vi "program seq..vi"(6 "IOList":T3, 7 "Cluster data":T5, 11 "Filepath":path=path "E:/My Project/2018-2019/Under development/Minda Ind. Switch -ID 144-145/Project/data/trail pro -12.txt") -> (0 "Error Out":errorcluster)   [LabVIEW 2015]
uses:
  Control PB/Active.ctl
  Control PB/deactive.ctl
  Control PB/output control.ctl
  Control PB/input control.ctl
  Control PB/timer.ctl
  Control PB/Remove list.ctl
  Control Button/Exit.ctl
  Control PB/Add_s.ctl
  Control PB/Delete_.ctl
  Control Button/Save.ctl
  Control PB/motor.ctl
  Control PB/Camera.ctl
  Control PB/Barcode.ctl
  Galobal variable_TI.vi
panel:
  in  "CAN":bool
  in  "Feature Step edit":bool
  out "Step List 4":string[](array[string])
  out "Step List 3":string[](array[string])
  in  "Barcode":T1
  in  "Camera":T2
  out "x <= y?":bool
  out "Cancel":bool
  out "Step List 2":string[](array[string])
  out "Pokayoka Result":cluster{"Sensor Name":string, "Boolean":bool}[](array[cluster])
  in  "Feed Back Channel":i32[](listbox)=[0]
  out "Input":bool[](array[boolean])
  out "Feature List (Out) 2":T4(array[cluster])
  out "error out 2":errorcluster
  in  "Control":bool
  out "Station No":string
  out "Model Name":string
  out "Model":string
  in  "Motor":T6
  in  "Feature List":i32(listbox) caption="Steps List"
  in  "Deletefeature list":T7
  in  "Add feature list":T8
  in  "Deactive":T9
  in  "Active":T10
  in  "Program step":i32(listbox)
  in  "Remove Step":T11
  in  "Wait Time":u32=100 caption="Timer(ms)" max=600000 step=1
  in  "Timer":T12
  in  "Save":T13
  in  "stop":T14
  in  "op Add":T15
  in  "Input Add":T16
  out "Step List":string[](array[string])
  out "output cluster":T17
  in  "Analog":bool
  in  "Analog Input":i32[](listbox)=[0]
  in  "Control Channel":i32[](listbox)=[7]
  in  "Steps":T18(array[cluster])
  in  "Program mode":string="Data"
  out "error out":errorcluster
  out "Feature List (Out)":T19(array[cluster])
  # "Program Sequence Window"
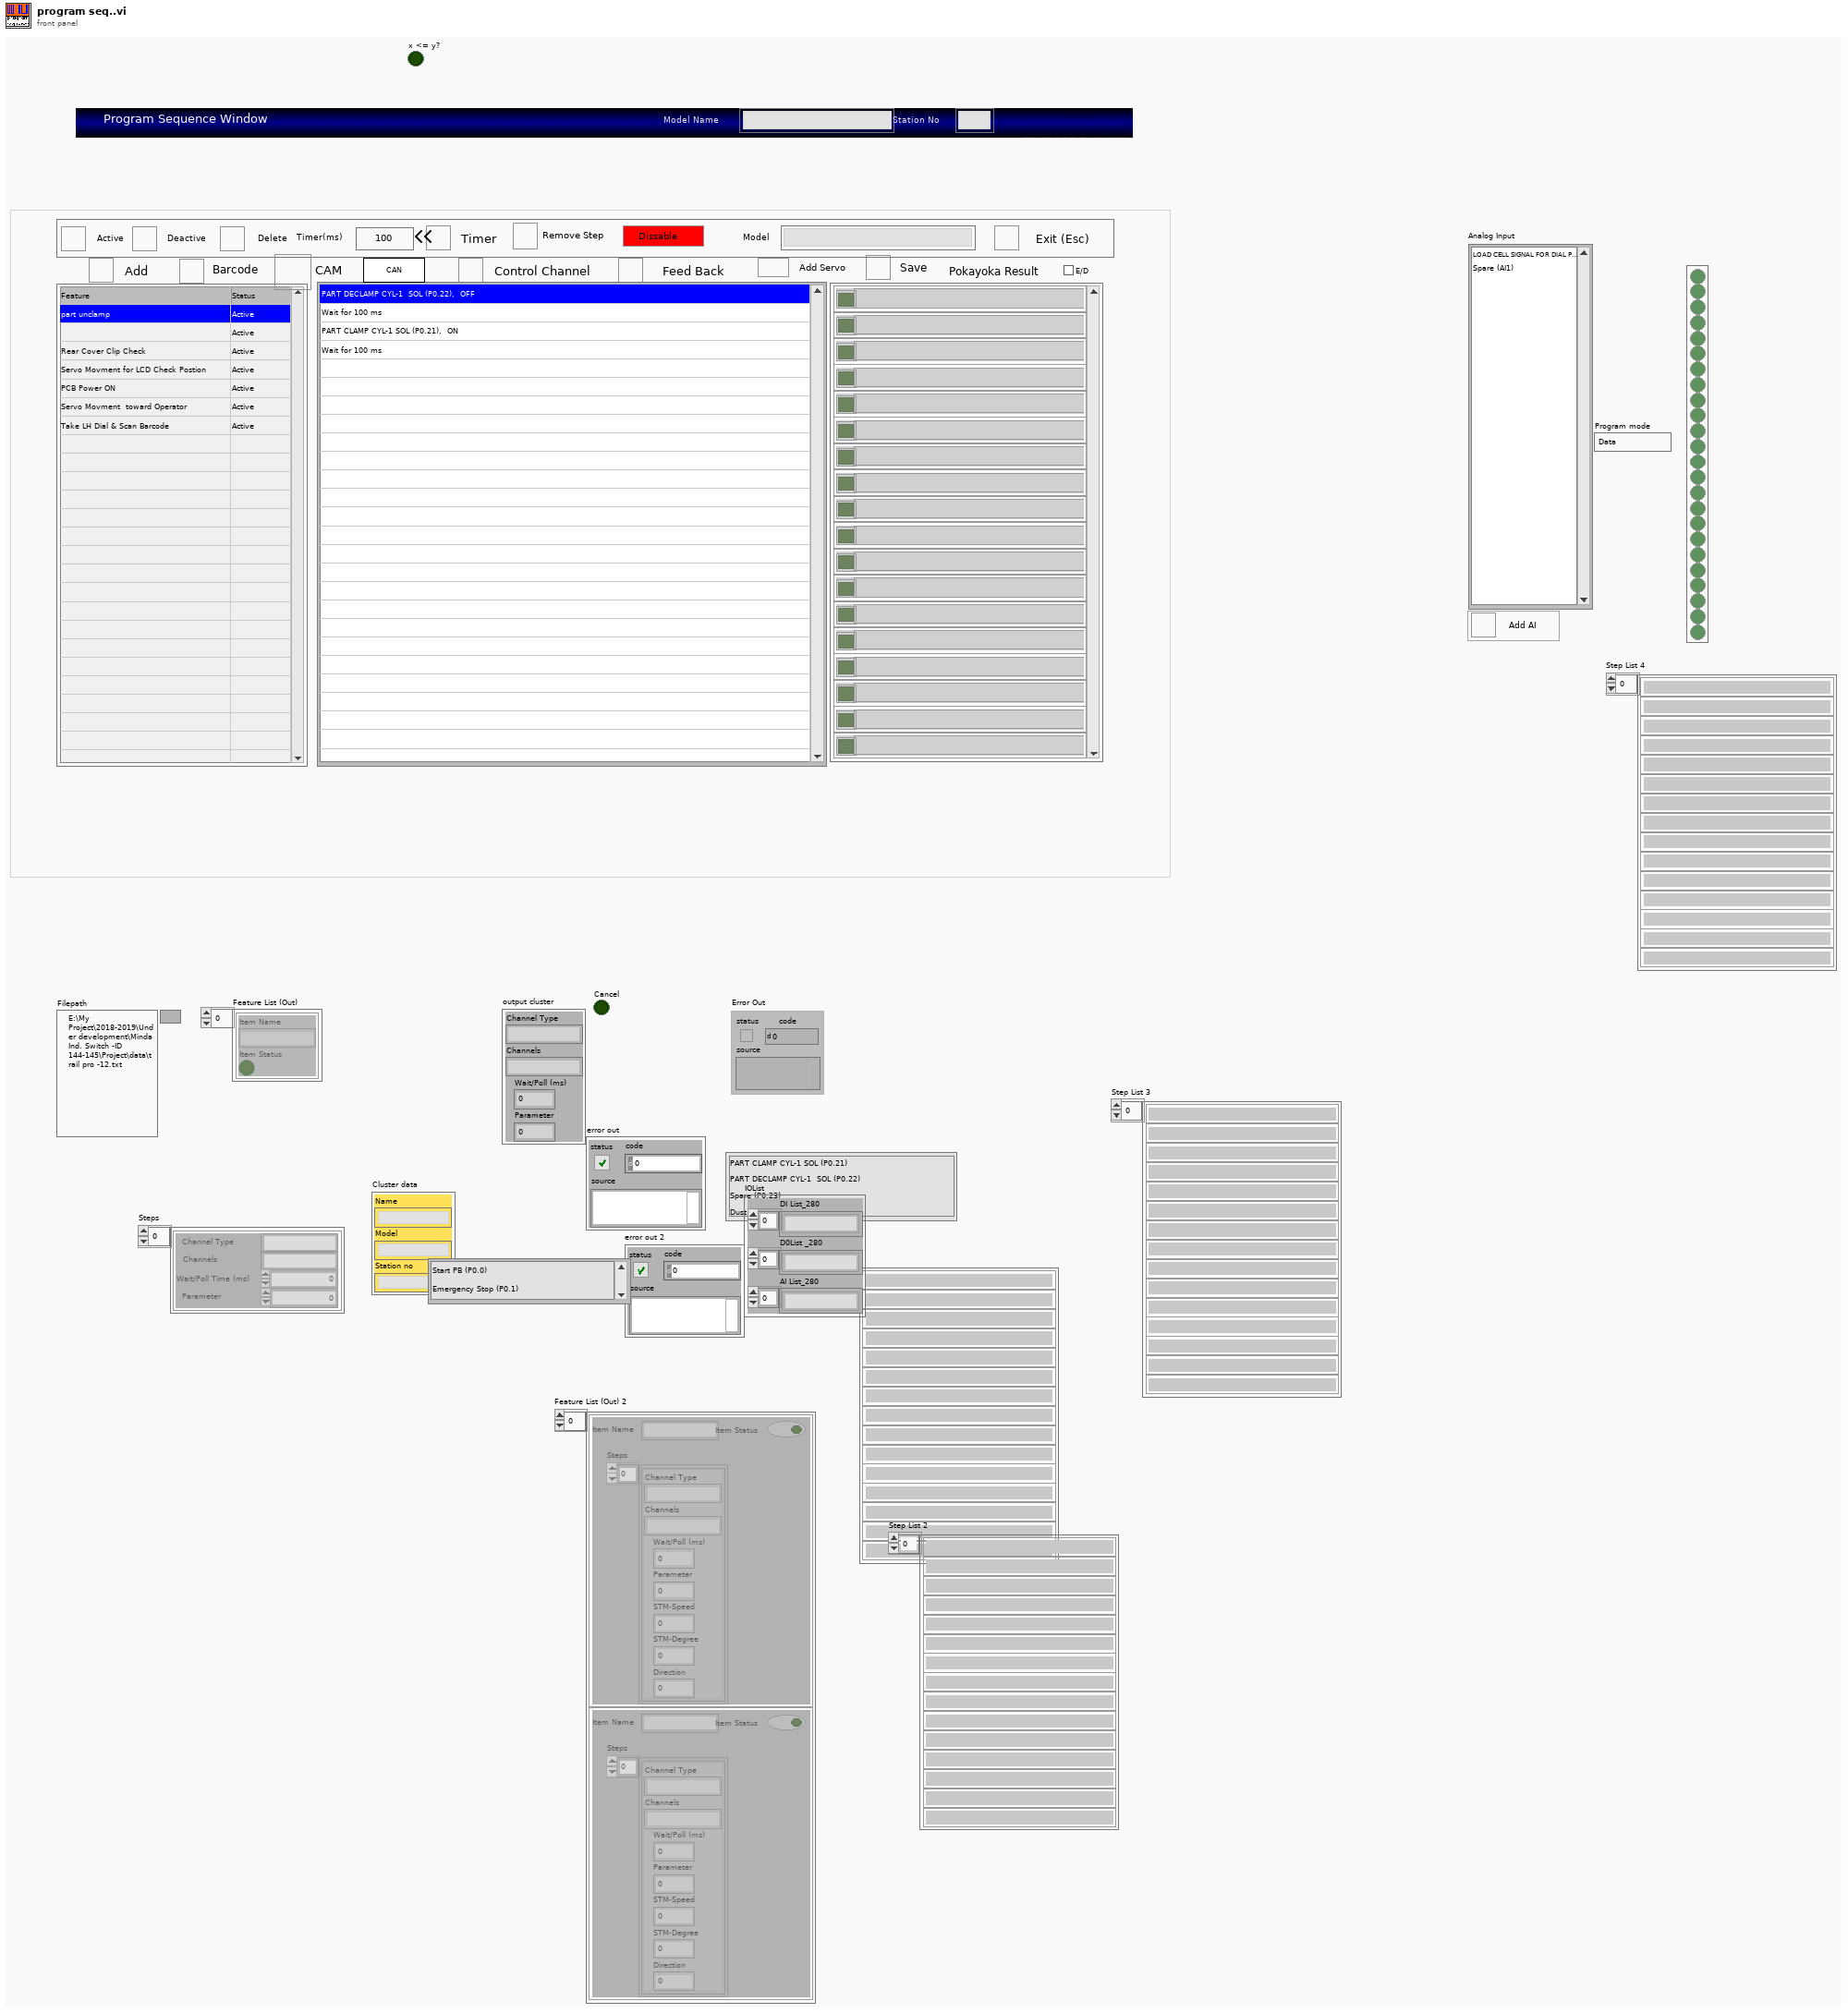
[diagram p1: front panel]
types:
  T1 = typedef "Barcode.ctl" = bool
  T2 = typedef "Camera.ctl" = bool
  T3 = cluster{"DI List_280":string[], "D0List _280":string[], "AI List_280":string[]}
  T4 = cluster{"Item Name":string, "Item Status":bool, "Steps":cluster{"Channel Type":string, "Channels":string, "Wait/Poll (ms)":u32, "Parameter":u8, "STM-Speed":i32, "STM-Degree":u32, "Direction":u8}[]}[]
  T5 = cluster{"Name":string, "Model":string, "Station no":string}
  T6 = typedef "motor.ctl" = bool
  T7 = typedef "Delete_.ctl" = bool
  T8 = typedef "Add_s.ctl" = bool
  T9 = typedef "deactive.ctl" = bool
  T10 = typedef "Active.ctl" = bool
  T11 = typedef "Remove list.ctl" = bool
  T12 = typedef "timer.ctl" = bool
  T13 = typedef "Save.ctl" = bool
  T14 = typedef "Exit.ctl" = bool
  T15 = typedef "output control.ctl" = bool
  T16 = typedef "input control.ctl" = bool
  T17 = cluster{"Channel Type":string, "Channels":string, "Wait/Poll (ms)":u32, "Parameter":u8}
  T18 = cluster{"Channel Type":string, "Channels":string, "Wait/Poll Time (ms)":u32, "Parameter":u8}[]
  T19 = cluster{"Item Name":string, "Item Status":bool}[]
  T20 = cluster{"Channel Type":string, "Channels":string, "Wait/Poll (ms)":u32, "Parameter":u8, "STM-Speed":i32, "STM-Degree":i32, "Direction":u8}
  T21 = cluster{"Item Name":string, "Item Status":bool, "Steps":cluster{"Channel Type":string, "Channels":string, "Wait/Poll (ms)":u32, "Parameter":u8, "STM-Speed":i32, "STM-Degree":u32, "Direction":u8}[]}
  T22 = cluster{"Channel Type":string, "Channels":string, "Wait/Poll (ms)":u32, "Parameter":u8, "STM-Speed":i32, "STM-Degree":u32, "Direction":u8}[]
  T23 = cluster{"Item Name":string, "Active":T10, "Steps":cluster{"Channel Type":string, "Channels":string, "Wait/Poll (ms)":u32, "Parameter":u8, "STM-Speed":i32, "STM-Degree":u32, "Direction":u8}[]}
  T24 = cluster{"Channel Type":string, "Channels":string, "Wait/Poll (ms)":u32, "Parameter":u8, "STM-Speed":i32, "STM-Degree":i32, "Direction":u8}[]
  T25 = cluster{"Feature name ":string, bool, cluster{"Channel Type":string, "Channels":string, "Wait/Poll (ms)":u32, "Parameter":u8, "STM-Speed":i32, "STM-Degree":i32, "Direction":u8}[]}
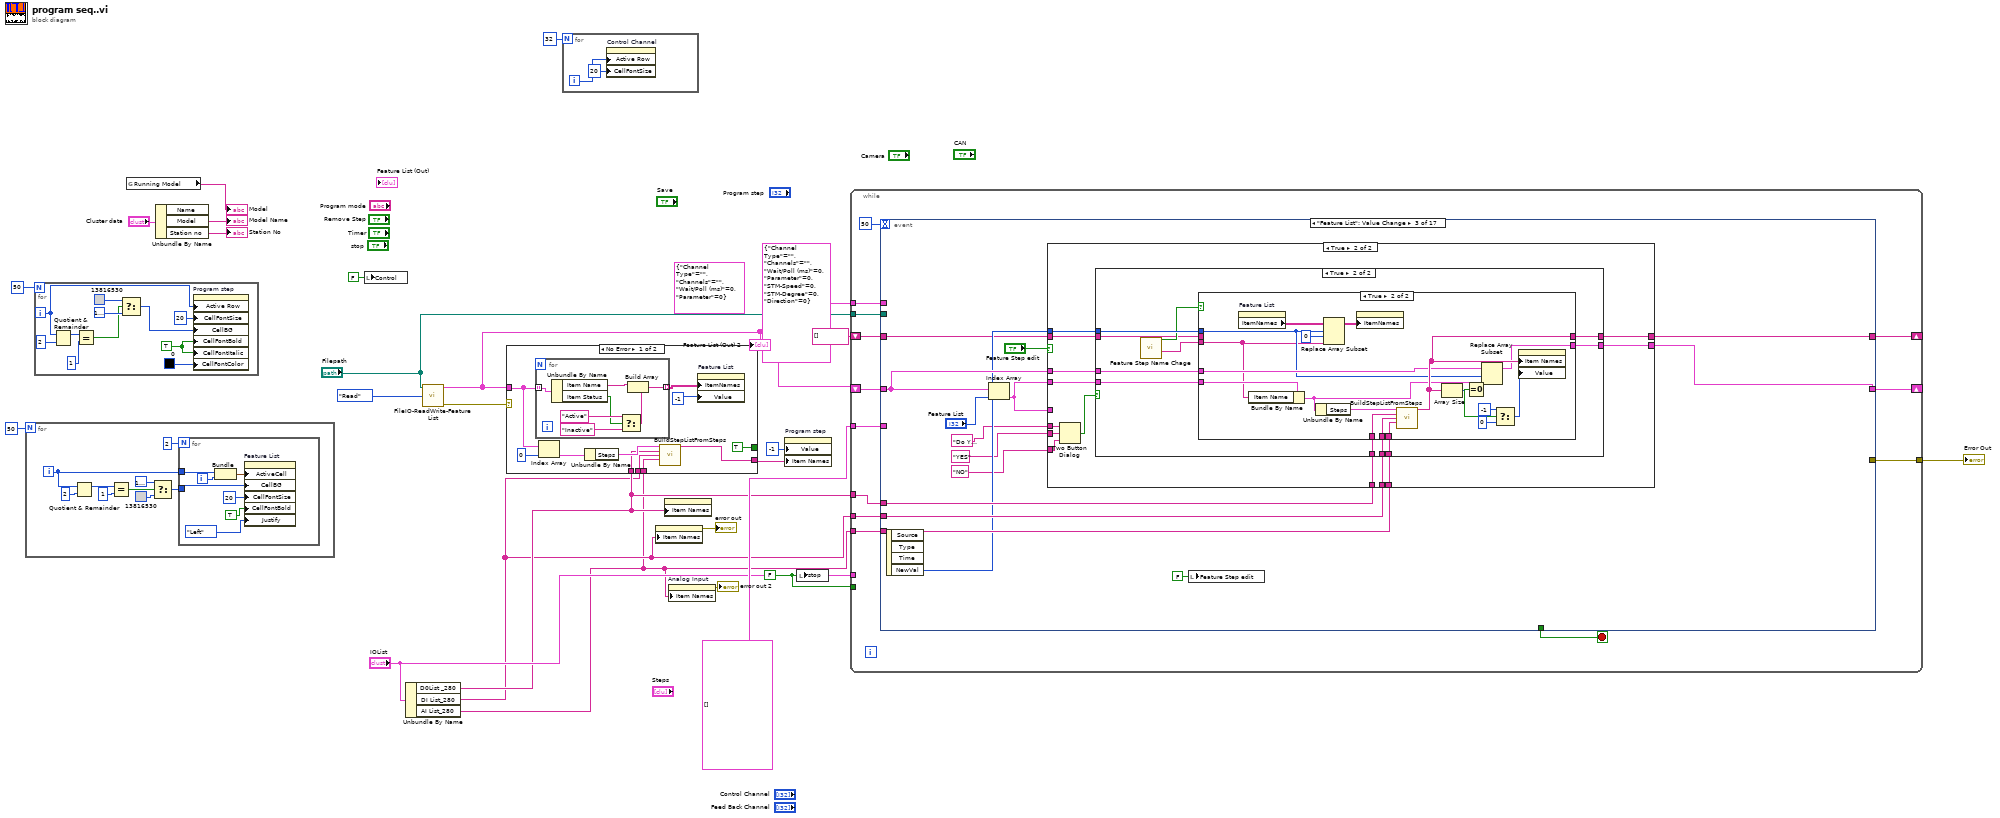
[diagram p0: block diagram]
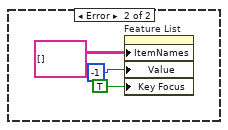
[diagram p2: hidden frame]
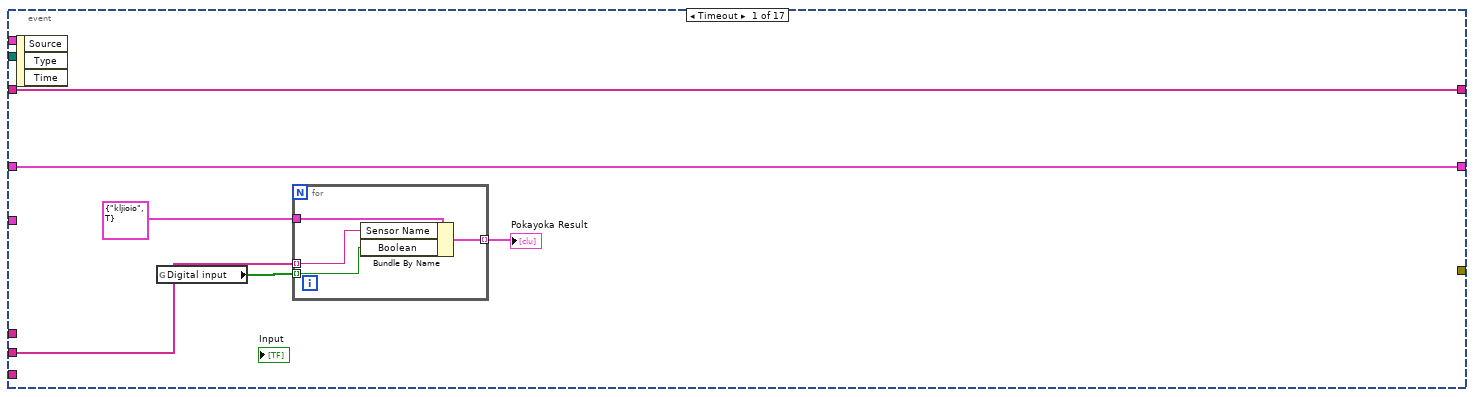
[diagram p3: hidden frame]
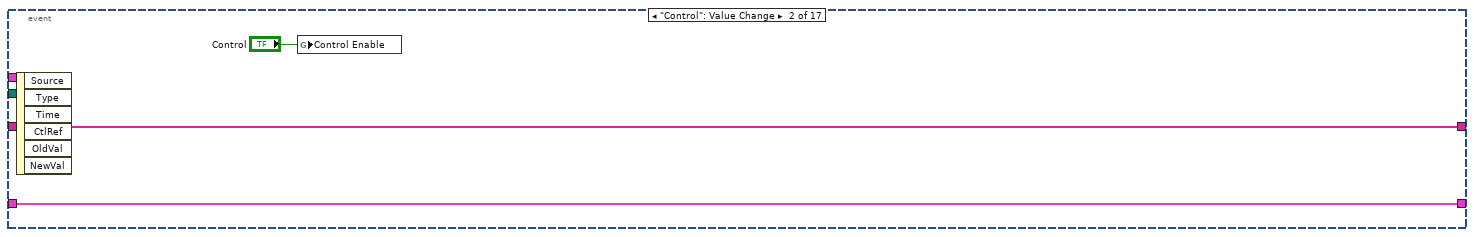
[diagram p4: hidden frame]
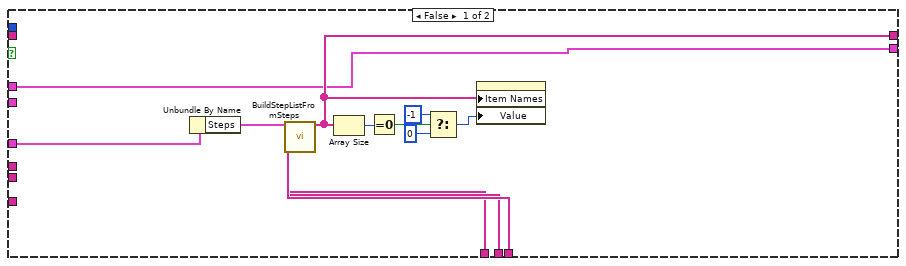
[diagram p5: hidden frame]
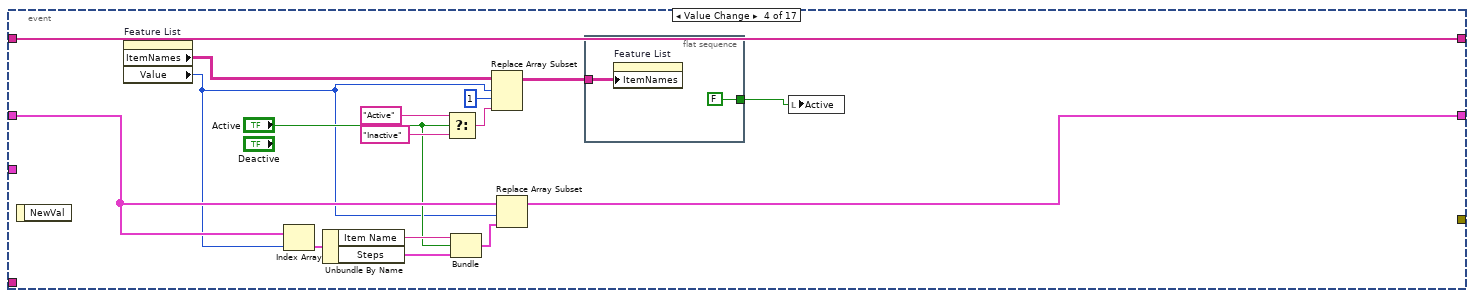
[diagram p8: hidden frame]
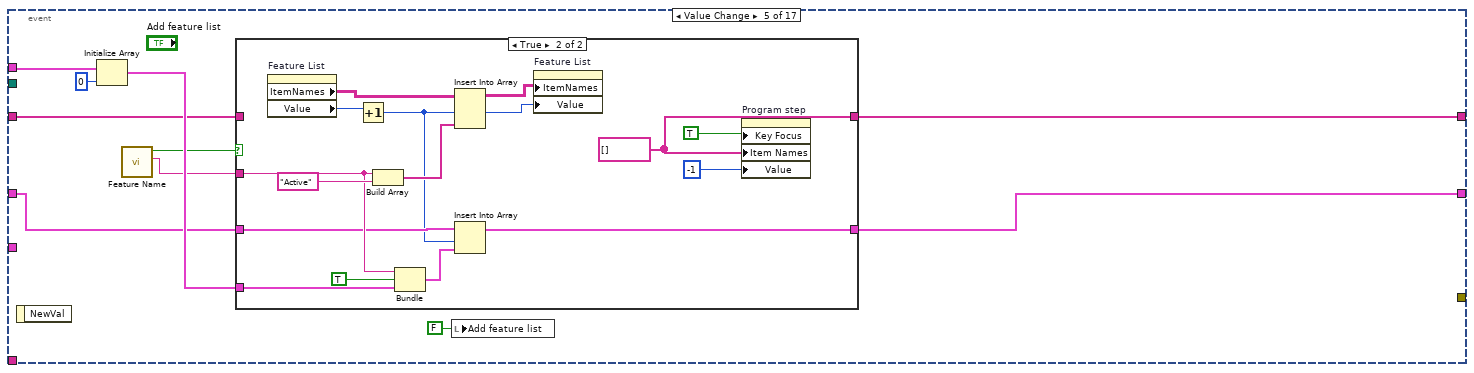
[diagram p9: hidden frame]
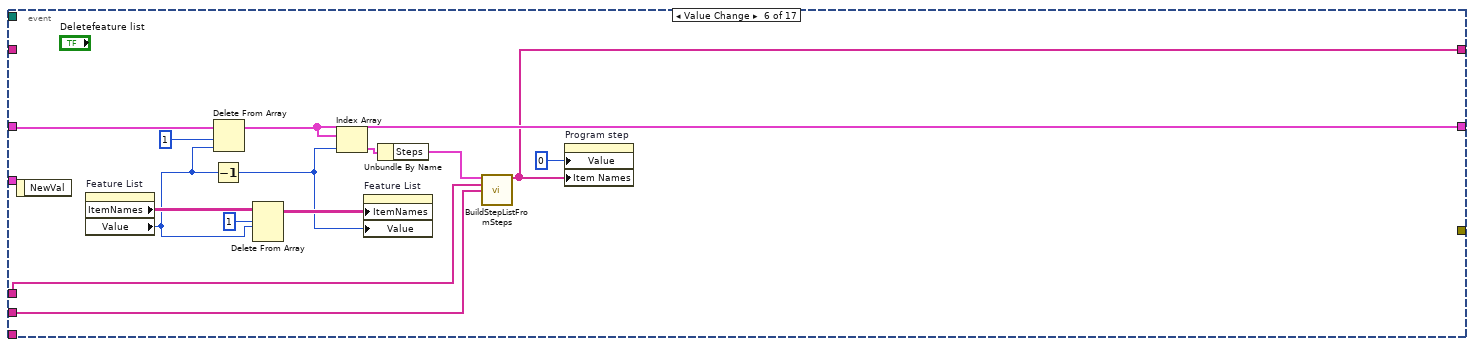
[diagram p11: hidden frame]
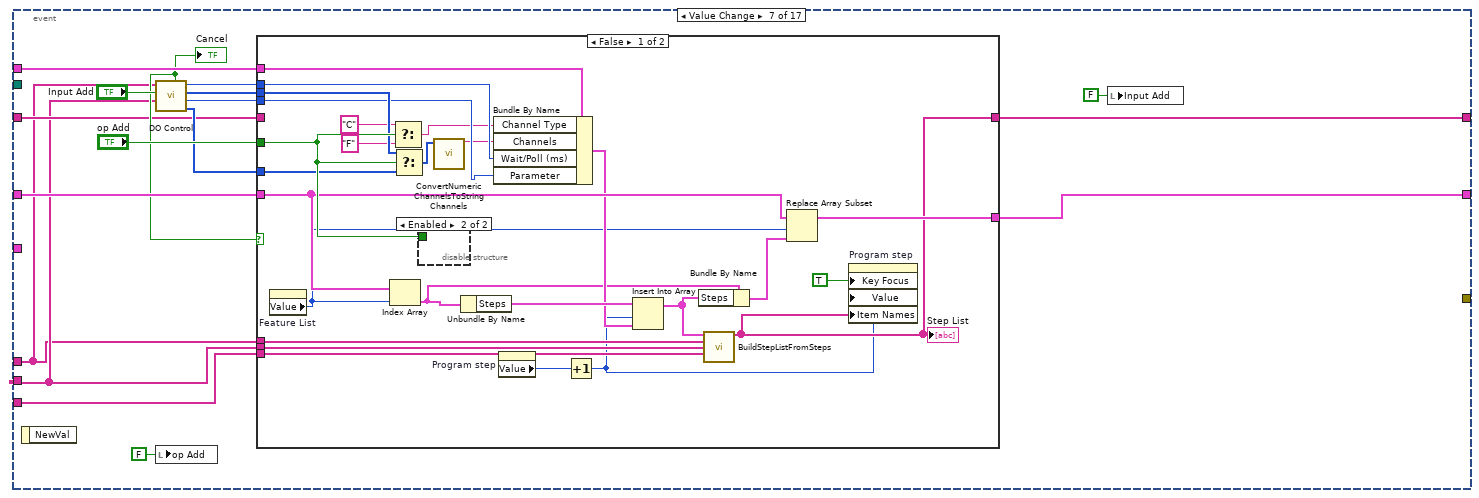
[diagram p12: hidden frame]
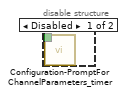
[diagram p13: hidden frame]
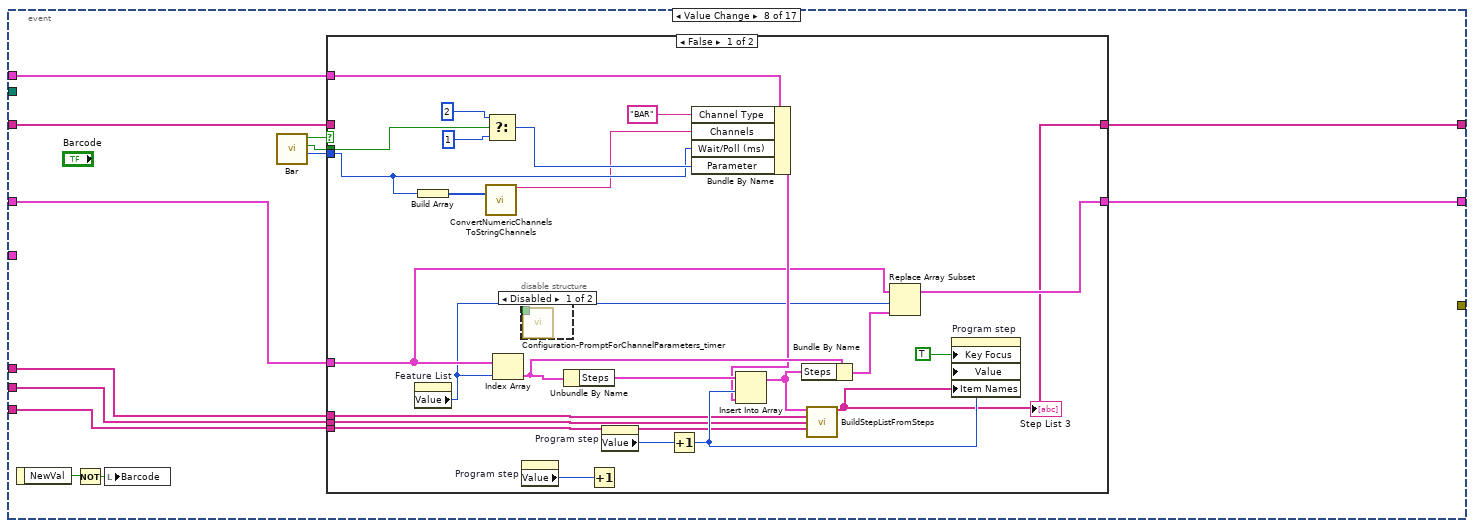
[diagram p15: hidden frame]
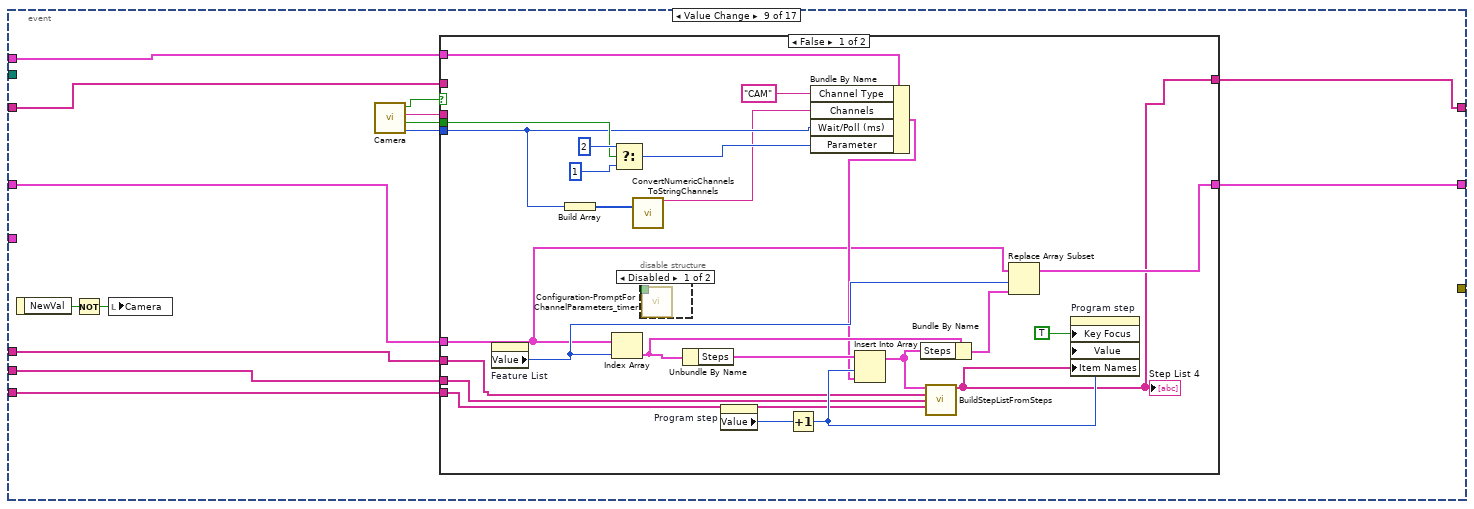
[diagram p18: hidden frame]
diagram:
  w9 = FALSE ("stop")
  (unwired) T17 {"Channel Type"="", "Channels"="", "Wait/Poll (ms)"=0, "Parameter"=0} ("Step")
  n1 = for {
    N: 50 -> [_]
    i -> [w33]
    n2 = Quotient & Remainder(x=w33, y=2) -> (x-y*floor(x/y)=w31:i32)  [unwired: 1 out]
    n3 = Equal?(x=w31, y=1) -> (x = y?=w29:bool)
    n4 = Select(t=u32 16777225 ("Color Box"), s=w29, f=u32 13816530 ("Color Box")) -> (s? t:f=w26:u32)
    n5 = for {
      N: 2 -> [_]
      tunnel: w33 -> [w41]
      tunnel: w26 -> [w38]
      i -> [w40]
      n6 = Bundle(w41, w40) -> (w39:cluster{i32, i32})  [unwired: 1 in]
      n7 = property on="Feature List" class="MCListbox (strict)"("ActiveCell"=w39, "CellBG"=w38, "CellFontSize"=u32 20 ("Active Cell:Cell Font:Size"), "CellFontBold"=TRUE ("Active Cell:Cell Font:Bold"), "Justify"=enum16{"Left", "Center", "Right"}."Left" ("Active Cell:Cell Justification")) -> ()  [unwired: 2 in, 2 out]
    }
  }
  n8 = for {
    N: 50 -> [_]
    i -> [w46]
    w43 = TRUE
    n9 = Quotient & Remainder(x=w46, y=2) -> (x-y*floor(x/y)=w49:i32)  [unwired: 1 out]
    n10 = Equal?(x=w49, y=1) -> (x = y?=w47:bool)
    n11 = Select(t=u32 13816530 ("Color Box"), s=w47, f=u32 16777226 ("Color Box")) -> (s? t:f=w44:u32)
    n12 = property on="Program step" class="LstBox (strict)"("Active Row"=w46, "CellFontSize"=u32 20 ("Active Row:Cell Font:Size"), "CellBG"=w44, "CellFontBold"=w43, "CellFontItalic"=w43, "CellFontColor"=u32 0 ("Color Box")) -> ()  [unwired: 2 in, 2 out]
  }
  n13 = global read "Galobal variable_TI.vi" "Running Model"() -> (→"Model":string)
  n14 = Unbundle By Name("Cluster data") -> ("Model"=→"Model Name":string, "Station no"=→"Station No":string)  [unwired: 1 out]
  n15 = local write "Control"(FALSE ("Control")) -> ()
  n16 = Unbundle By Name("IOList") -> ("D0List _280"=w5:string[], "DI List_280"=w4:string[], "AI List_280"=w3:string[])
  n17 = call "FileIO-ReadWrite-FeatureList.vi"("Filepath"="Filepath", "Read/Write"=enum16{"Read", "Write"}."Read") -> ("Feature List (Out)"=w16:T4, "Error Out"=w20:errorcluster)  [unwired: 12 in]
  "Feature List (Out) 2" <- w16
  n18 = case shown="No Error" w20 {
    tunnel: w16 -> [w63 _]
    tunnel: w5 -> [w59 _]
    tunnel: w4 -> [w58 _]
    tunnel: w3 -> [w57 _]
    tunnel: [w56 _] -> w19
    tunnel: [TRUE ("Key Focus") _] -> _
    frame No Error {
      n19 = for {
        tunnel: w63 -> [w70] mode=indexing
        tunnel: [w64] -> w54 mode=indexing
        n20 = Unbundle By Name(w70) -> ("Item Name"=w66:string, "Item Status"=w67:bool)
        n21 = Select(t="Active", s=w67, f="Inactive") -> (s? t:f=w65:string)
        n22 = Build Array(w66, w65) -> (w64:string[])
      }
      n23 = Index Array(array=w63, index=0) -> (element=w61:T21)
      n24 = Unbundle By Name(w61) -> ("Steps"=w60:T22)
      n25 = call "BuildStepListFromSteps.vi"("Steps"=w60, "Control Channels"=w59, "Feedback Channels"=w58, "AI"=w57) -> ("Step List"=w56:string[])  [unwired: 11 in]
      n26 = property on="Feature List" class="MCListbox (strict)"("ItemNames"=w54, "Value"=-1 ("Feautre list")) -> ()  [unwired: 2 in, 2 out]
    }
    frame Error {
      n27 = property on="Feature List" class="MCListbox (strict)"("ItemNames"=string[][] [] ("Item Names"), "Value"=-1 ("Feautre list"), "Key Focus"=TRUE) -> ()  [unwired: 2 in, 2 out]
    }
  }
  n28 = for {
    N: 32 -> [_]
    i -> [w75]
    n29 = property on="Control Channel" class="LstBox (strict)"("Active Row"=w75, "CellFontSize"=u32 20 ("Active Row:Cell Font:Size")) -> ()  [unwired: 2 in, 2 out]
  }
  n30 = property on="Feed Back Channel" class="LstBox (strict)"("Item Names"=w4) -> (error out=→"error out":errorcluster)  [unwired: 2 in, 1 out]
  n31 = property on="Control Channel" class="LstBox (strict)"("Item Names"=w5) -> ()  [unwired: 2 in, 2 out]
  n32 = property on="Analog Input" class="LstBox (strict)"("Item Names"=w3) -> (error out=→"error out 2":errorcluster)  [unwired: 2 in, 1 out]
  n33 = property on="Program step" class="LstBox (strict)"("Value"=-1 ("Step feautre list"), "Item Names"=w19) -> ()  [unwired: 2 in, 2 out]
  n34 = local write "stop"(w9) -> ()
  n35 = while {
    shift-right: [w86] -> _
    shift-left: w16 -> [w77]
    tunnel: T20 {"Channel Type"="", "Channels"="", "Wait/Poll (ms)"=0, "Parameter"=0, "STM-Speed"=0, "STM-Degree"=0, "Direction"=0} ("Step") -> [w87]
    shift-right: [w85] -> _
    shift-left: string[] [] ("Step List") -> [w84]
    tunnel: w5 -> [w83]
    tunnel: w4 -> [w82]
    tunnel: [w81] -> w23
    tunnel: w3 -> [w80]
    tunnel: T4 [] ("Feature List (Out) 2") -> [w79]
    tunnel: "Filepath" -> [w78]
    tunnel: w9 -> [_]
    tunnel: "IOList" -> [_]
    stop <- w88 stop-if-true
    n36 = event shown="[2] \"Feature List\": Value Change" {
      selector: _ -> [_ _ _ _ _ _ _ _ _ _ _ _ _ _ _ _ _]
      dyn-events: _ -> [_ _ _ _ _ _ _ _ _ _ _ _ _ _ _ _ _]
      timeout: 50 -> [_ _ _ _ _ _ _ _ _ _ _ _ _ _ _ _ _]
      tunnel: [_ _ _ _ _ _ _ _ _ _ _ _ _ _ TRUE ("stop") _ TRUE ("Discard?")] -> w88
      tunnel: w77 -> [w94 w100 w110 w183 w200 w232 w248 w288 w331 w372 w402 w423 w445 w454 w514 w536 w613]
      tunnel: w87 -> [_ _ _ _ w203 _ w251 w293 w335 w379 w407 w432 _ _ _ w537 _]
      tunnel: [w94 w100 w109 w181 w199 w231 w249 w287 w330 w367 w394 w422 w444 w456 w514 w532 w613] -> w86
      tunnel: [w93 w101 w116 w180 w196 w226 w247 w286 w329 w366 w393 w419 w439 w471 w513 w531 w614] -> w85
      tunnel: w84 -> [w93 w101 w102 w180 w195 _ w238 w281 w325 _ _ _ _ _ w513 w530 w614]
      tunnel: w83 -> [_ _ w115 _ _ w228 w236 w289 w332 w369 w399 w421 w441 w473 _ w533 _]
      tunnel: w82 -> [w92 _ w114 _ _ w227 w237 w290 w333 w370 w398 w420 w440 w472 _ w534 _]
      tunnel: [_ _ _ _ _ _ _ _ _ _ _ _ _ w464 _ _ _] -> w81
      tunnel: w80 -> [_ _ w113 _ _ _ w246 w291 w334 w371 w397 w418 _ w465 _ w535 _]
      tunnel: w79 -> [_ _ _ _ _ _ _ _ _ _ _ _ _ w470 _ _ _]
      tunnel: w78 -> [_ _ _ _ _ _ _ _ _ _ _ _ _ w455 _ _ _]
      event Timeout {
        n37 = event-data() -> ()  [unwired: 1 in, 3 out]
        n38 = global read "Galobal variable_TI.vi" "Digital input"() -> (w89:bool[])
        n39 = for {
          tunnel: w92 -> [w97] mode=indexing
          tunnel: cluster{"Sensor Name":string, "Boolean":bool} {"Sensor Name"="kljioio", "Boolean"=TRUE} ("Cluster") -> [w98]
          tunnel: [w96] -> w90 mode=indexing
          tunnel: w89 -> [w95] mode=indexing
          n40 = Bundle By Name(cluster=w98, "Sensor Name"=w97, "Boolean"=w95) -> (w96:cluster{"Sensor Name":string, "Boolean":bool})
        }
        "Pokayoka Result" <- w90
      }
      event "Control": Value Change {
        n41 = event-data() -> ()  [unwired: 1 in, 6 out]
        n42 = global write "Galobal variable_TI.vi" "Control Enable"("Control") -> ()
      }
      event "Feature List": Value Change {
        n43 = event-data() -> ("NewVal"=w108:i32)  [unwired: 1 in, 3 out]
        n44 = Index Array(array=w110, index="Feature List") -> (element=w107:T21)
        n45 = case shown="True" "Feature Step edit" {
          tunnel: w107 -> [w124 _]
          tunnel: [w118 w138] -> w116
          tunnel: w115 -> [w121 w139]
          tunnel: w114 -> [w122 w141]
          tunnel: w113 -> [w123 w140]
          tunnel: w110 -> [w117 w137]
          tunnel: [w117 w134] -> w109
          tunnel: w108 -> [_ w136]
          tunnel: w107 -> [_ w135]
          tunnel: "Do You Want Change The Feature List Name?" -> [_ w132]
          tunnel: "YES" -> [_ w131]
          tunnel: "NO" -> [_ w130]
          tunnel: w102 -> [_ w129]
          frame False {
            n46 = Unbundle By Name(w124) -> ("Steps"=w128:T22)
            n47 = call "BuildStepListFromSteps.vi"("Steps"=w128, "Control Channels"=w121, "Feedback Channels"=w122, "AI"=w123) -> ("Step List"=w118:string[])  [unwired: 11 in]
            n48 = Array Size(array=w118) -> (size(s)=w126:i32)
            n49 = Equal To 0?(x=w126) -> (x = 0?=w127:bool)
            n50 = Select(t=-1 ("Step List"), s=w127, f=0 ("Step List")) -> (s? t:f=w119:i32)
            n51 = property on="Program step" class="LstBox (strict)"("Item Names"=w118, "Value"=w119) -> ()  [unwired: 2 in, 2 out]
          }
          frame True {
            n52 = Two Button Dialog(message=w132, 1:w130, 2:w131) -> (T button?=w133:bool)
            n53 = case shown="True" w133 {
              tunnel: w141 -> [_ w154]
              tunnel: w140 -> [_ w153]
              tunnel: w139 -> [_ w152]
              tunnel: [w142 w151] -> w138
              tunnel: w137 -> [w143 w150]
              tunnel: w136 -> [_ w149]
              tunnel: w135 -> [_ w148]
              tunnel: [w143 w147] -> w134
              tunnel: w129 -> [w142 w144]
              frame False {
              }
              frame True {
                n54 = call "Feature Step Name Chage.vi"() -> ("Feature Step Nameout"=w146:string, "Next"=w145:bool)  [unwired: 10 in]
                n55 = case shown="True" w145 {
                  tunnel: w154 -> [_ w171]
                  tunnel: w153 -> [_ w170]
                  tunnel: w152 -> [_ w168]
                  tunnel: [w156 w167] -> w151
                  tunnel: w150 -> [w155 w163]
                  tunnel: w149 -> [_ w161]
                  tunnel: w148 -> [_ w160]
                  tunnel: [w155 w158] -> w147
                  tunnel: w146 -> [_ w157]
                  tunnel: w144 -> [w156 _]
                  frame False {
                  }
                  frame True {
                    n56 = property on="Feature List" class="MCListbox (strict)"() -> ("ItemNames"=w166:string[][])  [unwired: 2 in, 2 out]
                    n57 = Bundle By Name(cluster=w160, "Item Name"=w157) -> (w159:T21)
                    n58 = Unbundle By Name(w159) -> ("Steps"=w162:T22)
                    n59 = Replace Array Subset(array=w166, new element=w157, index (row)=w161, index (col)=0 ("disabled index (col)")) -> (w164:string[][])
                    n60 = property on="Feature List" class="MCListbox (strict)"("ItemNames"=w164) -> ()  [unwired: 2 in, 2 out]
                    n61 = call "BuildStepListFromSteps.vi"("Steps"=w162, "Control Channels"=w168, "Feedback Channels"=w171, "AI"=w170) -> ("Step List"=w167:string[])  [unwired: 11 in]
                    n62 = Array Size(array=w167) -> (size(s)=w173:i32)
                    n63 = Equal To 0?(x=w173) -> (x = 0?=w175:bool)
                    n64 = Replace Array Subset(array=w163, new element=w159, index=w161) -> (w158:T4)
                    n65 = Select(t=-1 ("Step List"), s=w175, f=0 ("Step List")) -> (s? t:f=w169:i32)
                    n66 = property on="Program step" class="LstBox (strict)"("Item Names"=w167, "Value"=w169) -> ()  [unwired: 2 in, 2 out]
                  }
                }
              }
            }
          }
        }
        n67 = local write "Feature Step edit"(FALSE ("Feature Step edit")) -> ()
      }
      event Value Change {
        n68 = event-data() -> ()  [unwired: 1 in, 1 out]
        n69 = property on="Feature List" class="MCListbox (strict)"() -> ("ItemNames"=w179:string[][], "Value"=w177:i32)  [unwired: 2 in, 2 out]
        n70 = Index Array(array=w183, index=w177) -> (element=w189:T21)
        n71 = Unbundle By Name(w189) -> ("Item Name"=w190:string, "Steps"=w191:T22)
        n72 = Select(t="Active", s="Active", f="Inactive" ("element")) -> (s? t:f=w186:string)
        n73 = Bundle("Item Name"=w190, "Active"="Active", "Steps"=w191) -> (w188:T23)  [unwired: 1 in]
        n74 = Replace Array Subset(array=w179, new element=w186, index (row)=w177, index (col)=1 ("disabled index (col)")) -> (w178:string[][])
        n75 = Replace Array Subset(array=w183, new element=w188, index=w177) -> (w181:T4)
        n76 = flat-sequence {
          tunnel: w178 -> [w193]
          tunnel: [T10 FALSE ("Active")] -> w176
          frame #0 {
            n77 = property on="Feature List" class="MCListbox (strict)"("ItemNames"=w193) -> ()  [unwired: 2 in, 2 out]
          }
        }
        n78 = local write "Active"(w176) -> ()
      }
      event Value Change {
        n79 = event-data() -> ()  [unwired: 1 in, 1 out]
        n80 = Initialize Array(w203, 0 ("dimension size")) -> (w201:T24)
        n81 = call "Feature Name.vi"() -> ("Feature name"=w197:string, "Out"=w198:bool)  [unwired: 10 in]
        n82 = case shown="True" w198 {
          tunnel: w201 -> [_ w219]
          tunnel: w200 -> [w205 w214]
          tunnel: [w205 w216] -> w199
          tunnel: w197 -> [_ w215]
          tunnel: [w204 w212] -> w196
          tunnel: w195 -> [w204 _]
          frame False {
          }
          frame True {
            w212 = string[] [] ("Item Names")
            n83 = property on="Feature List" class="MCListbox (strict)"() -> ("ItemNames"=w209:string[][], "Value"=w206:i32)  [unwired: 2 in, 2 out]
            n84 = Increment(x=w206) -> (x+1=w207:i32)
            n85 = Build Array(w215, "Active") -> (w210:string[])
            n86 = Bundle("Feature name"=w215, TRUE, w219) -> (w217:T25)  [unwired: 1 in]
            n87 = Insert Into Array(array=w209, index (row)=w207, new element=w210) -> (w208:string[][])  [unwired: 1 in]
            n88 = Insert Into Array(array=w214, index=w207, new element=w217) -> (w216:T4)
            n89 = property on="Feature List" class="MCListbox (strict)"("ItemNames"=w208, "Value"=w207) -> ()  [unwired: 2 in, 2 out]
            n90 = property on="Program step" class="LstBox (strict)"("Key Focus"=TRUE, "Item Names"=w212, "Value"=-1 ("Step feautre list")) -> ()  [unwired: 2 in, 2 out]
          }
        }
        n91 = local write "Add feature list"(FALSE ("Add feature list")) -> ()
      }
      event Value Change {
        n92 = event-data() -> ()  [unwired: 1 in, 1 out]
        n93 = property on="Feature List" class="MCListbox (strict)"() -> ("ItemNames"=w224:string[][], "Value"=w223:i32)  [unwired: 2 in, 2 out]
        n94 = Decrement(x=w223) -> (x-1=w221:i32)
        n95 = Delete From Array(array=w232, length=1, index=w223) -> (array with subset deleted=w231:T4)  [unwired: 1 out]
        n96 = Delete From Array(array=w224, length=1, index (row)=w223) -> (array with subset deleted=w222:string[][])  [unwired: 1 in, 1 out]
        n97 = Index Array(array=w231, index=w221) -> (element=w230:T21)
        n98 = property on="Feature List" class="MCListbox (strict)"("ItemNames"=w222, "Value"=w221) -> ()  [unwired: 2 in, 2 out]
        n99 = Unbundle By Name(w230) -> ("Steps"=w229:T22)
        n100 = call "BuildStepListFromSteps.vi"("Steps"=w229, "Control Channels"=w228, "Feedback Channels"=w227) -> ("Step List"=w226:string[])  [unwired: 12 in]
        n101 = property on="Program step" class="LstBox (strict)"("Value"=0 ("Step feautre list"), "Item Names"=w226) -> ()  [unwired: 2 in, 2 out]
      }
      event Value Change {
        n102 = event-data() -> ()  [unwired: 1 in, 1 out]
        n103 = call "DO Control.vi"("DI List_280"=w237, "s"="Input Add", "Control"=w236) -> ("Feedback"=w241:i32[], "Parameter (Out)"=w243:u8, "Control Channel"=w245:i32[], "Poll Time (Out)"=w244:u32, "Cancel"=w239:bool)  [unwired: 3 in, 1 out]
        "Cancel" <- w239
        n104 = local write "op Add"(T15 FALSE ("op Add")) -> ()
        n105 = case shown="False" w239 {
          tunnel: w251 -> [w277 _]
          tunnel: "op Add" -> [w276 _]
          tunnel: [w275 w280] -> w249
          tunnel: w248 -> [w274 w280]
          tunnel: w236 -> [w273 _]
          tunnel: w237 -> [w272 _]
          tunnel: [w271 w279] -> w247
          tunnel: w246 -> [w270 _]
          tunnel: w245 -> [w269 _]
          tunnel: w244 -> [w268 _]
          tunnel: w243 -> [w267 _]
          tunnel: w241 -> [w266 _]
          tunnel: w238 -> [_ w279]
          frame False {
            n106 = property on="Feature List" class="MCListbox (strict)"() -> ("Value"=w252:i32)  [unwired: 2 in, 2 out]
            n107 = Index Array(array=w274, index=w252) -> (element=w258:T21)
            n108 = Select(t="C", s=w276, f="F") -> (s? t:f=w263:string)
            n109 = Select(t=w269, s=w276, f=w266) -> (s? t:f=w262:i32[])
            n110 = disable-structure shown="Enabled" {
              disable-tunnel: w276 -> [w278 _]
              frame Disabled {
                n111 = call "Configuration-PromptForChannelParameters_timer.vi"("Control/Feedback\n(Default: False = Feedback)"=w278) -> ()  [unwired: 13 in, 2 out]
              }
              frame Enabled {
              }
            }
            n112 = call "ConvertNumericChannelsToStringChannels.vi"("Channels (In)"=w262) -> ("Channels (A:B:C:D...) (Out)"=w261:string)  [unwired: 14 in]
            n113 = Unbundle By Name(w258) -> ("Steps"=w260:T22)
            n114 = Bundle By Name(cluster=w277, "Channel Type"=w263, "Channels"=w261, "Wait/Poll (ms)"=w268, "Parameter"=w267) -> (w259:T20)
            n115 = property on="Program step" class="LstBox (strict)"() -> ("Value"=w253:i32)  [unwired: 2 in, 2 out]
            n116 = Increment(x=w253) -> (x+1=w254:i32)
            n117 = Insert Into Array "Insert Into Array"(array=w260, index=w254, new element=w259) -> (w256:T22)
            n118 = Bundle By Name(cluster=w258, "Steps"=w256) -> (w257:T21)
            n119 = call "BuildStepListFromSteps.vi"("Steps"=w256, "Control Channels"=w273, "Feedback Channels"=w272, "AI"=w270) -> ("Step List"=w271:string[])  [unwired: 11 in]
            "Step List" <- w271
            n120 = Replace Array Subset(array=w274, new element=w257, index=w252) -> (w275:T4)
            n121 = property on="Program step" class="LstBox (strict)"("Key Focus"=TRUE, "Value"=w254, "Item Names"=w271) -> ()  [unwired: 2 in, 2 out]
          }
          frame True {
          }
        }
        n122 = local write "Input Add"(T16 FALSE ("Input Add")) -> ()
      }
      event Value Change {
        n123 = event-data() -> ("NewVal"=w284:T1)  [unwired: 1 in]
        n124 = Not(x=w284) -> (.not. x?=w283:T1)
        n125 = local write "Barcode"(w283) -> ()
        n126 = call "Bar.vi"() -> ("Time Out Value"=w285:u8, "Barcode Scane"=w292:bool, "Out"=w282:bool)  [unwired: 8 in, 1 out]
        n127 = case shown="False" w282 {
          tunnel: w293 -> [w318 _]
          tunnel: w292 -> [w316 _]
          tunnel: w291 -> [w303 _]
          tunnel: w290 -> [w302 _]
          tunnel: w289 -> [w301 _]
          tunnel: w288 -> [w300 w320]
          tunnel: [w299 w320] -> w287
          tunnel: [w298 w321] -> w286
          tunnel: w285 -> [w296 _]
          tunnel: w281 -> [_ w321]
          frame False {
            n128 = property on="Feature List" class="MCListbox (strict)"() -> ("Value"=w297:i32)  [unwired: 2 in, 2 out]
            n129 = Build Array(w296) -> (w295:u8[])
            n130 = call "ConvertNumericChannelsToStringChannels.vi"("Channels (In)"=w295) -> ("Channels (A:B:C:D...) (Out)"=w294:string)  [unwired: 14 in]
            n131 = Select(t=2, s=w316, f=1) -> (s? t:f=w313:i32)
            n132 = Index Array(array=w300, index=w297) -> (element=w311:T21)
            n133 = disable-structure shown="Disabled" {
              disable-tunnel: _ -> [w319 _]
              frame Disabled {
                n134 = call "Configuration-PromptForChannelParameters_timer.vi"("Control/Feedback\n(Default: False = Feedback)"=w319) -> ()  [unwired: 13 in, 2 out]
              }
              frame Enabled {
              }
            }
            n135 = property on="Program step" class="LstBox (strict)"() -> ("Value"=w305:i32)  [unwired: 2 in, 2 out]
            n136 = Unbundle By Name(w311) -> ("Steps"=w312:T22)
            n137 = Increment(x=w305) -> ()  [unwired: 1 out]
            n138 = property on="Program step" class="LstBox (strict)"() -> ("Value"=w306:i32)  [unwired: 2 in, 2 out]
            n139 = Increment(x=w306) -> (x+1=w307:i32)
            n140 = Bundle By Name(cluster=w318, "Channel Type"="BAR", "Channels"=w294, "Wait/Poll (ms)"=w296, "Parameter"=w313) -> (w304:T20)
            n141 = Insert Into Array "Insert Into Array"(array=w312, index=w307, new element=w304) -> (w309:T22)
            n142 = Bundle By Name(cluster=w311, "Steps"=w309) -> (w310:T21)
            n143 = call "BuildStepListFromSteps.vi"("Steps"=w309, "Control Channels"=w301, "Feedback Channels"=w302, "AI"=w303) -> ("Step List"=w298:string[])  [unwired: 11 in]
            "Step List 3" <- w298
            n144 = Replace Array Subset(array=w300, new element=w310, index=w297) -> (w299:T4)
            n145 = property on="Program step" class="LstBox (strict)"("Key Focus"=TRUE, "Value"=w307, "Item Names"=w298) -> ()  [unwired: 2 in, 2 out]
          }
          frame True {
          }
        }
      }
      event Value Change {
        n146 = event-data() -> ("NewVal"=w322:T2)  [unwired: 1 in]
        n147 = Not(x=w322) -> (.not. x?=w323:T2)
        n148 = local write "Camera"(w323) -> ()
        n149 = call "Camera.vi"() -> ("Time Out (ms) 2"=w327:u8, "Camera 2"=w326:bool, "Feature name"=w328:string, "Out"=w324:bool)  [unwired: 8 in]
        n150 = case shown="False" w324 {
          tunnel: w335 -> [w346 _]
          tunnel: w334 -> [w345 _]
          tunnel: w333 -> [w344 _]
          tunnel: w332 -> [w343 _]
          tunnel: w331 -> [w342 w361]
          tunnel: [w341 w361] -> w330
          tunnel: [w340 w362] -> w329
          tunnel: w328 -> [_ _]
          tunnel: w327 -> [w337 _]
          tunnel: w326 -> [w339 _]
          tunnel: w325 -> [_ w362]
          frame False {
            n151 = property on="Feature List" class="MCListbox (strict)"() -> ("Value"=w348:i32)  [unwired: 2 in, 2 out]
            n152 = Build Array(w337) -> (w338:u8[])
            n153 = Index Array(array=w342, index=w348) -> (element=w354:T21)
            n154 = Select(t=2, s=w339, f=1) -> (s? t:f=w356:i32)
            n155 = call "ConvertNumericChannelsToStringChannels.vi"("Channels (In)"=w338) -> ("Channels (A:B:C:D...) (Out)"=w336:string)  [unwired: 14 in]
            n156 = disable-structure shown="Disabled" {
              disable-tunnel: _ -> [w360 _]
              frame Disabled {
                n157 = call "Configuration-PromptForChannelParameters_timer.vi"("Control/Feedback\n(Default: False = Feedback)"=w360) -> ()  [unwired: 13 in, 2 out]
              }
              frame Enabled {
              }
            }
            n158 = Unbundle By Name(w354) -> ("Steps"=w355:T22)
            n159 = property on="Program step" class="LstBox (strict)"() -> ("Value"=w349:i32)  [unwired: 2 in, 2 out]
            n160 = Increment(x=w349) -> (x+1=w350:i32)
            n161 = Bundle By Name(cluster=w346, "Channel Type"="CAM", "Channels"=w336, "Wait/Poll (ms)"=w337, "Parameter"=w356) -> (w347:T20)
            n162 = Insert Into Array "Insert Into Array"(array=w355, index=w350, new element=w347) -> (w352:T22)
            n163 = Bundle By Name(cluster=w354, "Steps"=w352) -> (w353:T21)
            n164 = call "BuildStepListFromSteps.vi"("Steps"=w352, "Control Channels"=w343, "Feedback Channels"=w344, "AI"=w345) -> ("Step List"=w340:string[])  [unwired: 11 in]
            "Step List 4" <- w340
            n165 = Replace Array Subset(array=w342, new element=w353, index=w348) -> (w341:T4)
            n166 = property on="Program step" class="LstBox (strict)"("Key Focus"=TRUE, "Value"=w350, "Item Names"=w340) -> ()  [unwired: 2 in, 2 out]
          }
          frame True {
          }
        }
      }
      event "Analog": Value Change {
        n167 = event-data() -> ()  [unwired: 1 in, 1 out]
        n168 = property on="Feature List" class="MCListbox (strict)"() -> ("Value"=w363:i32)  [unwired: 2 in, 2 out]
        n169 = call "Configuration-PromptForChannelParameters_timer.vi"("Control/Feedback\n(Default: False = Feedback)"=FALSE ("Control/Feedback\n(Default: False = Feedback)")) -> ("Poll Time (Out)"=w383:u32, "Parameter (Out)"=w382:u8)  [unwired: 13 in]
        n170 = Select(t="AI", s="Analog", f="N") -> (s? t:f=w385:string)
        n171 = call "ConvertNumericChannelsToStringChannels.vi"("Channels (In)"="Analog Input") -> ("Channels (A:B:C:D...) (Out)"=w384:string)  [unwired: 14 in]
        n172 = property on="Program step" class="LstBox (strict)"() -> ("Value"=w373:i32)  [unwired: 2 in, 2 out]
        n173 = Bundle By Name(cluster=w379, "Channel Type"=w385, "Channels"=w384, "Wait/Poll (ms)"=w383, "Parameter"=w382) -> (w368:T20)
        n174 = Index Array(array=w372, index=w363) -> (element=w377:T21)
        n175 = Increment(x=w373) -> (x+1=w364:i32)
        n176 = Unbundle By Name(w377) -> ("Steps"=w378:T22)
        n177 = Insert Into Array(array=w378, index=w364, new element=w368) -> (w375:T22)
        n178 = Bundle By Name(cluster=w377, "Steps"=w375) -> (w376:T21)
        n179 = call "BuildStepListFromSteps.vi"("Steps"=w375, "Control Channels"=w369, "Feedback Channels"=w370, "AI"=w371) -> ("Step List"=w366:string[])  [unwired: 11 in]
        n180 = Replace Array Subset(array=w372, new element=w376, index=w363) -> (w367:T4)
        n181 = property on="Program step" class="LstBox (strict)"("Key Focus"=TRUE, "Value"=w364, "Item Names"=w366) -> ()  [unwired: 2 in, 2 out]
      }
      event Value Change {
        n182 = event-data() -> ()  [unwired: 1 in, 1 out]
        n183 = property on="Feature List" class="MCListbox (strict)"() -> ("Value"=w401:i32)  [unwired: 2 in, 2 out]
        n184 = property on="Program step" class="LstBox (strict)"() -> ("Value"=w400:i32)  [unwired: 2 in, 2 out]
        n185 = Select(t="STM", s="Motor", f="N") -> (s? t:f=w412:string)
        n186 = call "STM-program.vi"() -> ("OutDir"=w411:i32, "Out Speed"=w409:i32, "Out Degree"=w410:dbl, "Channels (A:B:C:D...) (Out)"=w389:string)  [unwired: 7 in, 1 out]
        n187 = Increment(x=w400) -> (x+1=w395:i32)
        n188 = Bundle By Name(cluster=w407, "Channel Type"=w412, "Channels"=w389, "Wait/Poll (ms)"=u32 0, "Parameter"=u8 0, "STM-Degree"=w410, "STM-Speed"=w409, "Direction"=w411) -> (w392:T20)
        n189 = Index Array(array=w402, index=w401) -> (element=w405:T21)
        n190 = Unbundle By Name(w405) -> ("Steps"=w406:T22)
        n191 = Insert Into Array(array=w406, index=w395, new element=w392) -> (w403:T22)
        n192 = Bundle By Name(cluster=w405, "Steps"=w403) -> (w404:T21)
        n193 = local write "Motor"(FALSE ("Motor")) -> ()
        n194 = call "BuildStepListFromSteps.vi"("Steps"=w403, "Control Channels"=w399, "Feedback Channels"=w398, "AI"=w397) -> ("Step List"=w393:string[])  [unwired: 11 in]
        n195 = Replace Array Subset(array=w402, new element=w404, index=w401) -> (w394:T4)
        n196 = property on="Program step" class="LstBox (strict)"("Key Focus"=TRUE, "Value"=w395, "Item Names"=w393) -> ()  [unwired: 2 in, 2 out]
      }
      event Value Change {
        n197 = event-data() -> ()  [unwired: 1 in, 1 out]
        n198 = property on="Feature List" class="MCListbox (strict)"() -> ("Value"=w415:i32)  [unwired: 2 in, 2 out]
        n199 = Index Array(array=w423, index=w415) -> (element=w426:T21)
        n200 = Bundle By Name(cluster=w432, "Channel Type"="N", "Wait/Poll (ms)"="Wait Time") -> (w428:T20)
        n201 = Unbundle By Name(w426) -> ("Steps"=w427:T22)
        n202 = property on="Program step" class="LstBox (strict)"() -> ("Value"=w429:i32)  [unwired: 2 in, 2 out]
        n203 = Increment(x=w429) -> (x+1=w416:i32)
        n204 = Insert Into Array(array=w427, index=w416, new element=w428) -> (w424:T22)
        n205 = Bundle By Name(cluster=w426, "Steps"=w424) -> (w425:T21)
        n206 = call "BuildStepListFromSteps.vi"("Steps"=w424, "Control Channels"=w421, "Feedback Channels"=w420, "AI"=w418) -> ("Step List"=w419:string[])  [unwired: 11 in]
        n207 = property on="Program step" class="LstBox (strict)"("Item Names"=w419, "Value"=w416, "Key Focus"=TRUE) -> ()  [unwired: 2 in, 2 out]
        n208 = Replace Array Subset(array=w423, new element=w425, index=w415) -> (w422:T4)
      }
      event Value Change {
        n209 = event-data() -> ()  [unwired: 1 in, 2 out]
        n210 = property on="Feature List" class="MCListbox (strict)"() -> ("Value"=w434:i32)  [unwired: 2 in, 2 out]
        n211 = Index Array(array=w445, index=w434) -> (element=w451:T21)
        n212 = property on="Program step" class="LstBox (strict)"() -> ("Value"=w433:i32)  [unwired: 2 in, 2 out]
        n213 = Unbundle By Name(w451) -> ("Item Name"=w449:string, "Item Status"=w448:bool, "Steps"=w447:T22)
        n214 = Equal?(x=w433, y=-1) -> (x = y?=w437:bool)
        n215 = Select(t=0 ("y"), s=w437, f=w433) -> (s? t:f=w435:i32)
        n216 = Delete From Array(array=w447, length=1, index=w435) -> (array with subset deleted=w443:T22)  [unwired: 1 out]
        n217 = Bundle("Item Name"=w449, "Item Status"=w448, "Steps"=w443) -> (w446:T21)  [unwired: 1 in]
        n218 = call "BuildStepListFromSteps.vi"("Steps"=w443, "Control Channels"=w441, "Feedback Channels"=w440) -> ("Step List"=w439:string[])  [unwired: 12 in]
        n219 = Replace Array Subset(array=w445, new element=w446, index=w434) -> (w444:T4)
        n220 = property on="Program step" class="LstBox (strict)"("Item Names"=w439, "Value"=w435, "Key Focus"=TRUE) -> ()  [unwired: 2 in, 2 out]
      }
      event Value Change {
        n221 = event-data() -> ()  [unwired: 1 in, 1 out]
        n222 = for {
          tunnel: w454 -> [w501] mode=indexing
          tunnel: [w496] -> w462 mode=indexing
          shift-right: [w495] -> w463
          shift-left: w470 -> [w498]
          n223 = Unbundle By Name(w501) -> ("Steps"=w502:T22, "Item Name"=w500:string, "Item Status"=w499:bool)
          n224 = Array Size(array=w502) -> (size(s)=w497:i32)
          n225 = case shown="Default" w497 {
            tunnel: w502 -> [_ w509]
            tunnel: w500 -> [_ w511]
            tunnel: w499 -> [_ w510]
            tunnel: [w504 w507] -> w495
            tunnel: w498 -> [w504 w505]
            tunnel: [FALSE TRUE] -> w496
            frame 0 {
            }
            frame Default {
              n226 = Bundle("Item Name"=w511, "Item Status"=w510, "Steps"=w509) -> (w506:T21)  [unwired: 1 in]
              n227 = Build Array (concatenate)(w505, w506) -> (w507:T4)
            }
          }
        }
        n228 = And Array Elements(Boolean array=w462) -> (logical AND=w461:bool)
        n229 = case shown="True" w461 {
          tunnel: [w474 w476] -> w456
          tunnel: w455 -> [_ w484]
          tunnel: [_ w482] -> w464
          tunnel: w463 -> [_ w477]
          tunnel: enum16{"Read", "Write"}."Write" ("Read/Write") -> [_ w483]
          tunnel: "Feature List successfully saved." -> [_ w481]
          tunnel: "Error in saving Feature List." -> [_ w480]
          tunnel: "Can't save Feature List as at least one feature doesn't have steps.\nPlease check." ("message") -> [w475 w479]
          tunnel: w454 -> [w474 _]
          frame False {
            n230 = One Button Dialog(message=w475) -> ()  [unwired: 1 in, 1 out]
          }
          frame True {
            n231 = call "FileIO-ReadWrite-FeatureList.vi"("Filepath"=w484, "Feature List (In)"=w477, "Read/Write"=w483) -> ("Feature List (Out)"=w476:T4, "Error Out"=w482:errorcluster)  [unwired: 11 in]
            n232 = case shown="Error" w482 {
              tunnel: w481 -> [w485 _]
              tunnel: w480 -> [_ w486]
              tunnel: w479 -> [_ _]
              tunnel: [w485 w486] -> w478
              frame No Error {
              }
              frame Error {
              }
            }
            n233 = One Button Dialog(message=w478) -> ()  [unwired: 1 in, 1 out]
          }
        }
        n234 = disable-structure shown="Enabled" {
          frame Disabled {
            n235 = call "Program seq path.vi"() -> ()  [unwired: 11 in, 1 out]
          }
          frame Enabled {
          }
        }
        n236 = Index Array(array=w456, index=0) -> (element=w468:T21)
        n237 = Unbundle By Name(w468) -> ("Steps"=w467:T22)
        n238 = for {
          tunnel: [w493] -> w453 mode=indexing
          tunnel: w456 -> [w488] mode=indexing
          tunnel: [w487] -> _
          i -> [w487]
          n239 = Unbundle By Name(w488) -> ("Item Name"=w494:string, "Item Status"=w492:bool)
          n240 = Select(t="Active", s=w492, f="Inactive") -> (s? t:f=w489:string)
          n241 = Build Array(w494, w489) -> (w493:string[])
        }
        n242 = call "BuildStepListFromSteps.vi"("Steps"=w467, "Control Channels"=w473, "Feedback Channels"=w472, "AI"=w465) -> ("Step List"=w471:string[])  [unwired: 11 in]
        n243 = property on="Program step" class="LstBox (strict)"("Item Names"=w471, "Value"=0 ("Step feautre list")) -> ()  [unwired: 2 in, 2 out]
        n244 = property on="Feature List" class="MCListbox (strict)"("ItemNames"=w453, "Value"=0 ("Feautre list")) -> ()  [unwired: 2 in, 2 out]
      }
      event Value Change {
        n245 = event-data() -> ()  [unwired: 1 in, 1 out]
      }
      event "Program step": Double Click {
        n246 = event-data() -> ("Row"=w528:i32)  [unwired: 1 in, 8 out]
        n247 = property on="Program step" class="LstBox (strict)"() -> ("Item Names"=w529:string[])  [unwired: 2 in, 2 out]
        n248 = Index Array(array=w529, index=w528) -> (element=w519:string)
        n249 = String Length(string=w519) -> (length=w518:i32)
        n250 = String Subset(string=w519, length (rest)=2 ("length (rest)")) -> (substring=w524:string)  [unwired: 1 in]
        n251 = String Subset(string=w519, length (rest)=4 ("length (rest)")) -> (substring=w522:string)  [unwired: 1 in]
        n252 = Less Or Equal?(x=w518, y=0) -> (x <= y?=w515:bool)
        "x <= y?" <- w515
        n253 = Equal?(x=w522, y="Wait") -> (x = y?=w520:bool)
        n254 = Equal?(x=w524, y="Ch") -> (x = y?=w525:bool)
        n255 = case shown="False" w515 {
          tunnel: w537 -> [w548 _]
          tunnel: w536 -> [w547 w611]
          tunnel: w535 -> [w546 _]
          tunnel: w534 -> [w545 _]
          tunnel: w533 -> [w544 _]
          tunnel: [w543 w611] -> w532
          tunnel: [w542 w612] -> w531
          tunnel: w530 -> [w541 w612]
          tunnel: w525 -> [w540 _]
          tunnel: w520 -> [w539 _]
          tunnel: enum32{"Output", "Input"}."Output" ("y") -> [w538 _]
          frame False {
            n256 = case shown="False" w539 {
              tunnel: w548 -> [w565 w598]
              tunnel: w547 -> [w564 w597]
              tunnel: w546 -> [w563 w601]
              tunnel: w545 -> [w562 w600]
              tunnel: w544 -> [w561 w599]
              tunnel: [w560 w596] -> w543
              tunnel: [w559 w595] -> w542
              tunnel: w541 -> [w553 _]
              tunnel: w540 -> [w552 _]
              tunnel: w538 -> [w550 _]
              frame False {
                n257 = call "DO Control.vi"("s"=w552) -> ("Feedback"=w555:i32[], "Parameter (Out)"=w556:u8, "Control Channel"=w558:i32[], "Poll Time (Out)"=w557:u32, "Tab Control 2"=w549:enum32{"Output", "Input"}, "Cancel"=w551:bool)  [unwired: 5 in]
                n258 = Equal?(x=w549, y=w550) -> (x = y?=w554:bool)
                n259 = case shown="False" w551 {
                  tunnel: w565 -> [w590 _]
                  tunnel: w564 -> [w589 w592]
                  tunnel: w563 -> [w588 _]
                  tunnel: w562 -> [w587 _]
                  tunnel: w561 -> [w586 _]
                  tunnel: [w585 w592] -> w560
                  tunnel: [w584 w593] -> w559
                  tunnel: w558 -> [w575 _]
                  tunnel: w557 -> [w574 _]
                  tunnel: w556 -> [w573 _]
                  tunnel: w555 -> [w572 _]
                  tunnel: w554 -> [w566 _]
                  tunnel: w553 -> [_ w593]
                  frame False {
                    n260 = property on="Feature List" class="MCListbox (strict)"() -> ("Value"=w576:i32)  [unwired: 2 in, 2 out]
                    n261 = Index Array(array=w589, index=w576) -> (element=w581:T21)
                    n262 = Select(t="C", s=w566, f="F") -> (s? t:f=w569:string)
                    n263 = Select(t=w575, s=w566, f=w572) -> (s? t:f=w568:i32[])
                    n264 = disable-structure shown="Disabled" {
                      disable-tunnel: w566 -> [w591 _]
                      frame Disabled {
                        n265 = call "Configuration-PromptForChannelParameters_timer.vi"("Control/Feedback\n(Default: False = Feedback)"=w591) -> ()  [unwired: 13 in, 2 out]
                      }
                      frame Enabled {
                      }
                    }
                    n266 = call "ConvertNumericChannelsToStringChannels.vi"("Channels (In)"=w568) -> ("Channels (A:B:C:D...) (Out)"=w567:string)  [unwired: 14 in]
                    n267 = Unbundle By Name(w581) -> ("Steps"=w583:T22)
                    n268 = Bundle By Name(cluster=w590, "Channel Type"=w569, "Channels"=w567, "Wait/Poll (ms)"=w574, "Parameter"=w573) -> (w582:T20)
                    n269 = property on="Program step" class="LstBox (strict)"() -> ("Value"=w577:i32)  [unwired: 2 in, 2 out]
                    n270 = Replace Array Subset(array=w583, new element=w582, index=w577) -> (w579:T22)
                    n271 = Bundle By Name(cluster=w581, "Steps"=w579) -> (w580:T21)
                    n272 = call "BuildStepListFromSteps.vi"("Steps"=w579, "Control Channels"=w586, "Feedback Channels"=w587, "AI"=w588) -> ("Step List"=w584:string[])  [unwired: 11 in]
                    "Step List 2" <- w584
                    n273 = Replace Array Subset(array=w589, new element=w580, index=w576) -> (w585:T4)
                    n274 = property on="Program step" class="LstBox (strict)"("Key Focus"=TRUE, "Value"=w577, "Item Names"=w584) -> ()  [unwired: 2 in, 2 out]
                  }
                  frame True {
                  }
                }
              }
              frame True {
                n275 = property on="Feature List" class="MCListbox (strict)"() -> ("Value"=w602:i32)  [unwired: 2 in, 2 out]
                n276 = call "Timer.vi"() -> ("Wait Time out"=w594:u32)  [unwired: 10 in, 1 out]
                n277 = Index Array(array=w597, index=w602) -> (element=w606:T21)
                n278 = Bundle By Name(cluster=w598, "Channel Type"="N", "Wait/Poll (ms)"=w594) -> (w608:T20)
                n279 = Unbundle By Name(w606) -> ("Steps"=w607:T22)
                n280 = property on="Program step" class="LstBox (strict)"() -> ("Value"=w609:i32)  [unwired: 2 in, 2 out]
                n281 = Replace Array Subset(array=w607, new element=w608, index=w609) -> (w604:T22)
                n282 = Bundle By Name(cluster=w606, "Steps"=w604) -> (w605:T21)
                n283 = call "BuildStepListFromSteps.vi"("Steps"=w604, "Control Channels"=w599, "Feedback Channels"=w600, "AI"=w601) -> ("Step List"=w595:string[])  [unwired: 11 in]
                n284 = property on="Program step" class="LstBox (strict)"("Item Names"=w595, "Value"=w609, "Key Focus"=TRUE) -> ()  [unwired: 2 in, 2 out]
                n285 = Replace Array Subset(array=w597, new element=w605, index=w602) -> (w596:T4)
              }
            }
          }
          frame True {
          }
        }
      }
      event Panel Close? {
        n286 = event-data() -> ()  [unwired: 1 in, 1 out]
        n287 = event-data("Discard?"=TRUE) -> ()  [unwired: 1 in, 1 out]
      }
    }
  }
  "Error Out" <- w23
